vi "camera.vi"(0 "Camera configuration":string="{\n\t\"type\": \"Camera\",\n\t\"listen_port\": 8010,\n\t\"location\": {\n\t\t\"x\": 0.0,\n\t\t\"y\": 0.0,\n\t\t\"z\": 250.0\n\t},\n\t\"rotation\": {\n\t\t\"pitch\": 0.0,\n\t\t\"yaw\": 0.0,\n\t\t\"roll\": 0.0\n\t},\n\t\"stream_dimensions\": {\n\t\t\"x\": 512.0,\n\t\t\"y\": 512.0\n\t},\n \"dynamic_range\": 1.0,\n \"fov\": 60.0,\n \"camera_matrix\": [\n      [433.0, 0.0,   256.0],\n      [0.0,   433.0, 256.0],\n      [0.0,   0.0,   1.0]\n  ],\t\n \"min_shutter\": 0.0005,\n \"max_shutter\": 0.0014,\n \"motion_blur_bias\": 0.1,\n \"white_balance\": 0.0,\n \"white_balance_temp_offset\": 0,\n \"exposure_compensation\": -1.0,\n \"image_noise_bias\": 0.05,\n\t\"ray_tracing\": {\n\t\t\"enable_ray_tracing\": false\n\t},\n\t\"color_filter_array\": {\n\t\t\"use_cfa\": false,\n\t\t\"cfa\": \"rccc\"\n\t},\n\t\"channels\": \"bgra\",\n\t\"viewport\": {\n\t\t\"enable_viewport\": false,\n\t\t\"fullscreen\": false,\n\t\t\"monitor_name\": \"\",\n\t\t\"monitor_number\": 0,\n\t\t\"window_offset\": {\n\t\t\t\"x\": 32,\n\t\t\t\"y\": 32\n\t\t},\n\t\t\"window_size\": {\n\t\t\t\"x\": 0,\n\t\t\t\"y\": 0\n\t\t}\n\t},\n\t\"annotation\": {\n\t\t\"include_annotation\": false,\n\t\t\"desired_tags\": [\n\t\t\t\"traffic_sign\", \"vehicle\"\n\t\t],\n\t\t\"include_lanes\": true,\n\t\t\"lane_sampling_distance\": 15000.0,\n\t\t\"lane_sampling_frequency\": 100.0,\n\t\t\"lane_subsampling\": 10.0,\n\t\t\"far_plane\": 10000.0,\n\t\t\"include_tags\": true,\n\t\t\"include_obb\": false,\n\t\t\"cull_partial_frame\": false,\n\t\t\"debug_draw\": false\n\t},\n\t\"max_distance\": 50000.0,\n\t\"channel_depth\": 1\n}", 3 "error In":errorcluster) -> (4 "Camera configuration":string, 6 "Image":picture, 7 "Raw data":u8[](array[numeric]), 8 "Annotation Data":string, 9 "error out":errorcluster)   [LabVIEW 2019, in "Lib_Simx.lvlib"]
doc: "Configures and reads the data stream for a RGB Camera sensor and outputs a picture with the specified format in the stream dimensions."
uses:
  Lib_Simx.lvlib
  controls/Header.ctl
  tools/simx_common.vi
panel:
  out "Header":T1 {"game_time" format="%_10g"}
  in  "Show Annotation":bool
  in  "null connection":refnum<k5>
  in  "camera_connection":refnum<k5>
  # "Note: set annotation settings in camera configuration json"
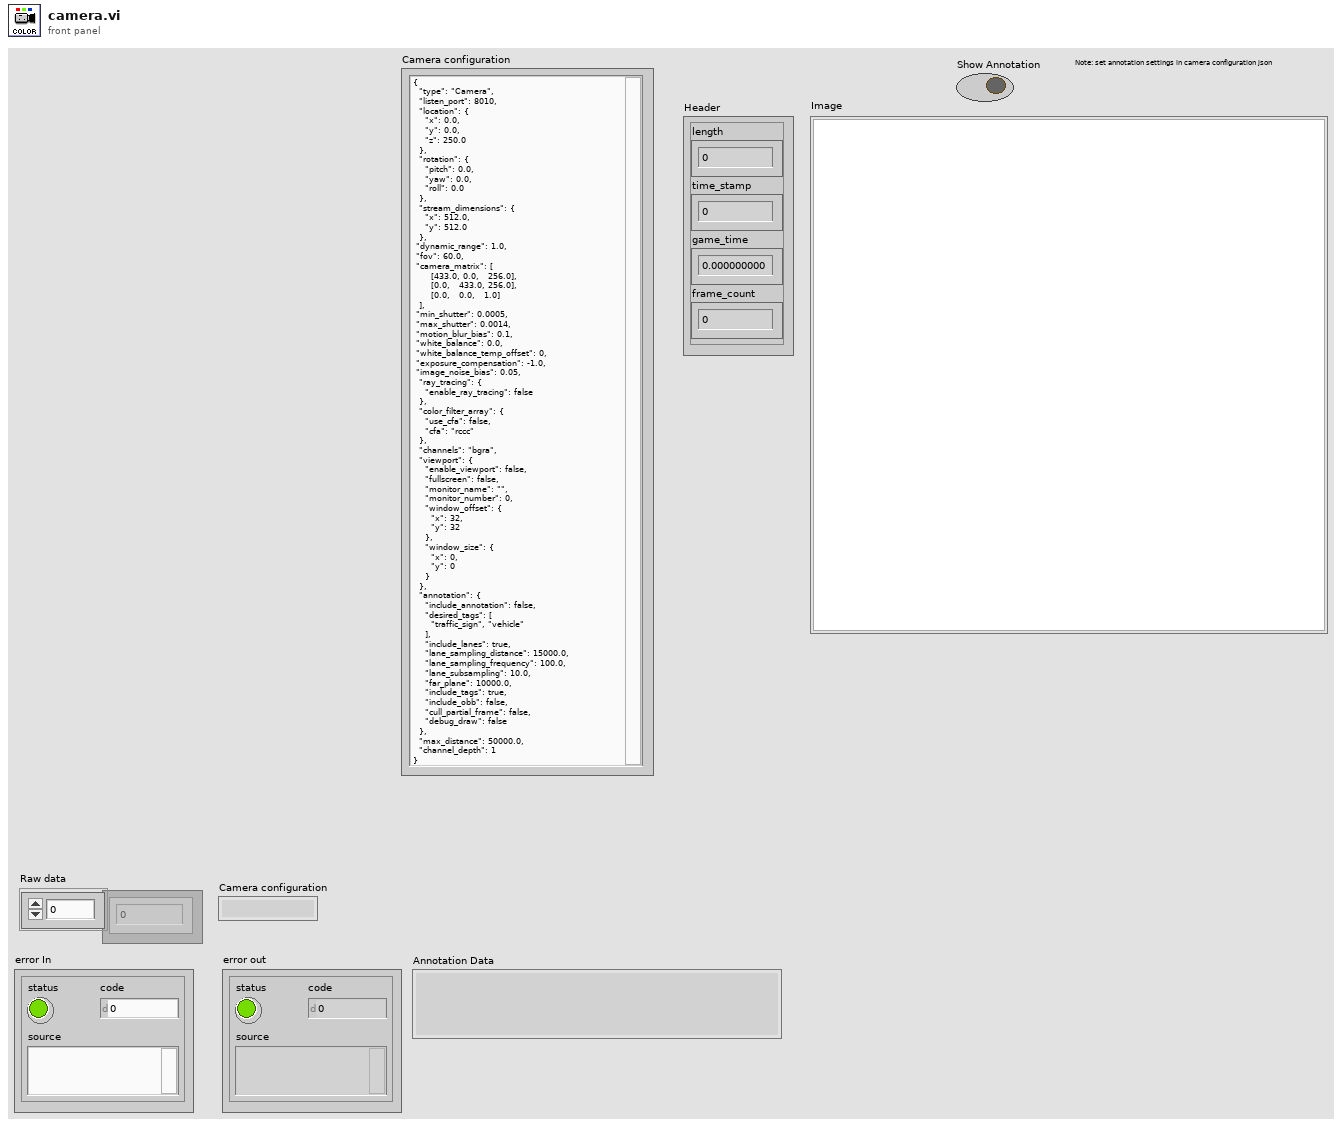
[diagram p1: front panel]
types:
  T1 = typedef "Lib_Simx.lvlib/Header.ctl" = cluster{"length":u32, "time_stamp":u32, "game_time":sgl, "frame_count":u32}
  T2 = typedef "Lib_Simx.lvlib/simx_connection.ctl" = cluster{"Config":T3, "Connections":T6, "Map":cluster{"lanes":cluster{"x":dbl[], "y":dbl[], "z":dbl[]}, "StartPosition":cluster{"start_points":T7, "StartRotation":dbl[], "StartLocation":dbl[]}, "Draw Map Size":T8, "DrawArea":cluster{"min_Y":dbl, "min_X":dbl, "Scale X":dbl, "Scale Y":dbl}, "Map":picture, "Map Geojson":string}}
  T3 = typedef "Lib_Simx.lvlib/config.ctl" = cluster{"Trajectory":T4, "Weather":T5}
  T4 = typedef "Lib_Simx.lvlib/trajectory.ctl" = cluster{"Number of frames":i32, "Frame number":i32, "Trajectory":string}
  T5 = typedef "Lib_Simx.lvlib/weather.ctl" = cluster{"id":string}
  T6 = typedef "Lib_Simx.lvlib/connections.ctl" = cluster{"Simulator Connection":refnum<k5>, "server_ip":string, "Port":i32, "Sensor connections":refnum<k5>[]}
  T7 = typedef "Lib_Simx.lvlib/start_points.ctl" = cluster{"locations":dbl[][], "rotations":dbl[][], "type":string[]}
  T8 = typedef "LVBoundsTypeDef.ctl" = cluster{"Width":u32, "Height":u32}
  T9 = typedef "Lib_Simx.lvlib/sensor_sample.ctl" = cluster{"Header":T1, "data out":string}
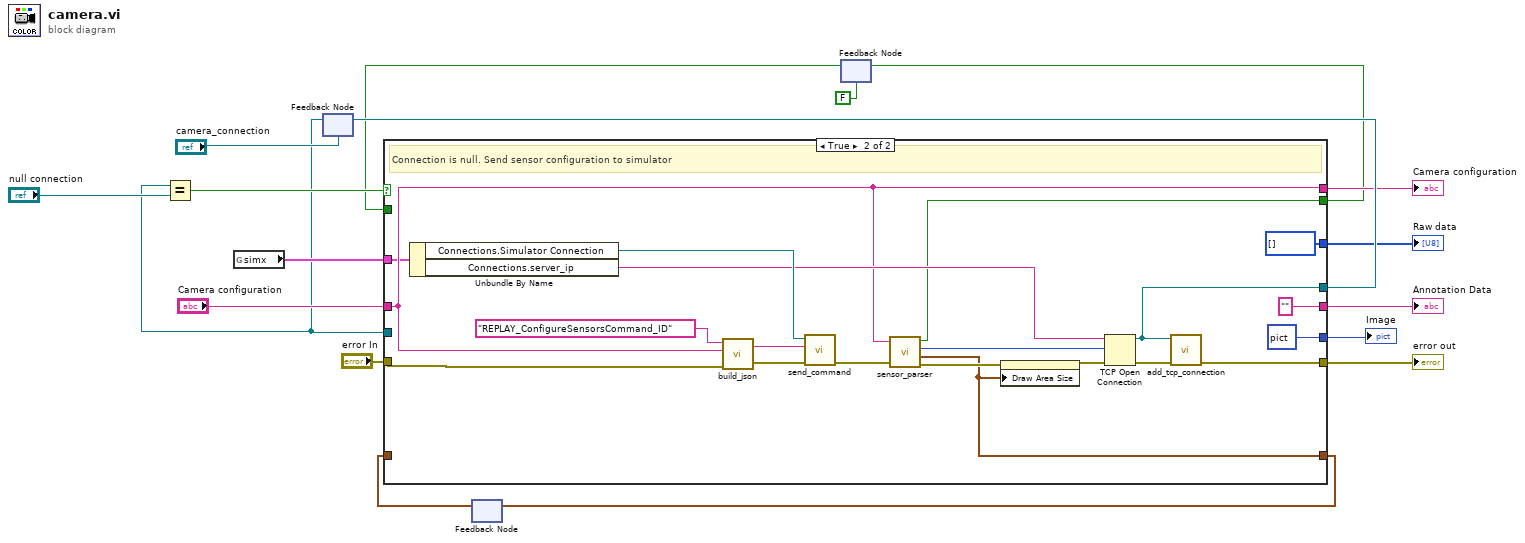
[diagram p0: block diagram]
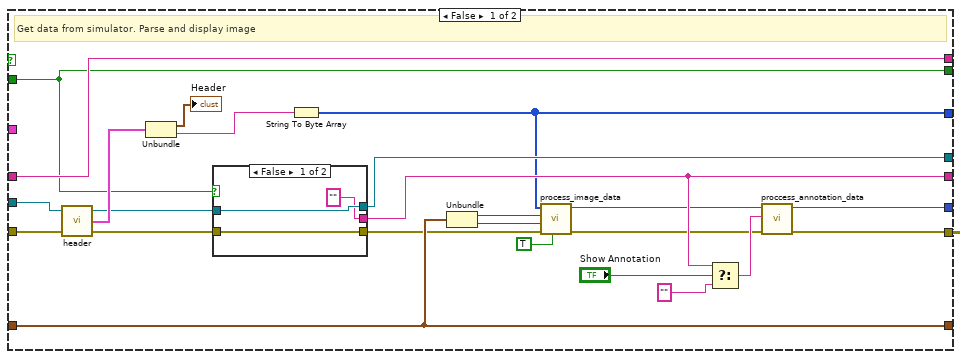
[diagram p2: hidden frame]
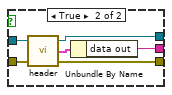
[diagram p3: hidden frame]
diagram:
  n1 = global read "simx_common.vi" "simx"() -> (w2:T2)
  n2 = feedback #1("camera_connection") -> (w1:refnum<k5>)
  n3 = Equal?(x=w1, y="null connection") -> (x = y?=w15:bool)
  n4 = feedback #2() -> (w10:cluster{"x dimension":i32, "y dimension":i32})  [unwired: 1 in]
  n5 = feedback #3(FALSE) -> (w4:bool)
  n6 = case shown="True" w15 {
    tunnel: [w35 w52] -> w13
    tunnel: "Camera configuration" -> [w37 w56]
    tunnel: [w27 w54] -> w16
    tunnel: w1 -> [w40 _]
    tunnel: "error In" -> [w39 w62]
    tunnel: w10 -> [w38 _]
    tunnel: [w34 picture data[5B] ("new picture")] -> w7
    tunnel: [w38 w59] -> w11
    tunnel: [w23 u8[] [] ("unsigned byte array")] -> w9
    tunnel: [w37 w56] -> w8
    tunnel: [w36 w58] -> w6
    tunnel: w4 -> [w36 _]
    tunnel: [w33 "" ("data out")] -> w3
    tunnel: w2 -> [_ w55]
    frame False {
      # "Get data from simulator. Parse and display image"
      n7 = call "header.vi"("error in"=w39, "TCP Network Connection in"=w40) -> ("error out"=w24:errorcluster, "Sensor sample"=w41:T9, "TCP Network Connection out"=w31:refnum<k5>)  [unwired: 1 in]
      n8 = Unbundle(w41) -> ("Header"=→"Header":T1, "data out"=w42:string)
      n9 = case shown="False" w36 {
        tunnel: w31 -> [w45 w51]
        tunnel: [w45 w50] -> w27
        tunnel: w24 -> [w43 w49]
        tunnel: ["" ("data out") w47] -> w33
        tunnel: [w43 w46] -> w26
        frame False {
        }
        frame True {
          n10 = call "header.vi"("error in"=w49, "TCP Network Connection in"=w51) -> ("error out"=w46:errorcluster, "Sensor sample"=w48:T9, "TCP Network Connection out"=w50:refnum<k5>)  [unwired: 1 in]
          n11 = Unbundle By Name(w48) -> ("data out"=w47:string)
        }
      }
      n12 = String To Byte Array(string=w42) -> (unsigned byte array=w23:u8[])
      n13 = Unbundle(w38) -> ("x dimension"=w22:i32, "y dimension"=w21:i32)
      n14 = call "process_image_data.vi"("RGBA"=TRUE, "error in"=w26, "y"=w21, "x"=w22, "Raw data"=w23) -> ("error out"=w25:errorcluster, "Image"=w20:picture)  [unwired: 3 in]
      n15 = Select(t=w33, s="Show Annotation", f="") -> (s? t:f=w28:string)
      n16 = call "proccess_annotation_data.vi"("error in"=w25, "Annotation Data"=w28, "Image in"=w20) -> ("error out"=w35:errorcluster, "Image out"=w34:picture)  [unwired: 2 in, 1 out]
    }
    frame True {
      # "Connection is null. Send sensor configuration to simulator"
      n17 = Unbundle By Name(w55) -> ("Connections.Simulator Connection"=w65:refnum<k5>, "Connections.server_ip"=w63:string)
      n18 = call "build_json.vi"("error in"=w62, "Message"=w56, "Command_ID"="REPLAY_ConfigureSensorsCommand_ID") -> ("error out"=w69:errorcluster, "JSON Out"=w70:string)  [unwired: 1 in]
      n19 = call "send_command.vi"("error in"=w69, "JSON Command"=w70, "TCP Network Connection in"=w65) -> ("error out"=w61:errorcluster)  [unwired: 1 in, 3 out]
      n20 = call "sensor_parser.vi"("Sensor configuration"=w56, "error in"=w61) -> ("include_annotation"=w58:bool, "Port out"=w57:u16, "Stream dimensions"=w59:cluster{"x dimension":i32, "y dimension":i32}, "error out"=w60:errorcluster)  [unwired: 1 in]
      n21 = property on="Image" class="Pict"(error in=w60, "Draw Area Size"=w59) -> (error out=w64:errorcluster)  [unwired: 1 in, 1 out]
      n22 = TCP Open Connection(address=w63, remote port or service name=w57, error in (no error)=w64) -> (connection ID=w54:refnum<k5>, error out=w53:errorcluster)  [unwired: 2 in]
      n23 = call "add_tcp_connection.vi"("error in"=w53, "Sensor connection"=w54) -> ("error out"=w52:errorcluster)  [unwired: 5 in]
    }
  }
  "error out" <- w13
  "Image" <- w7
  "Raw data" <- w9
  "Camera configuration" <- w8
  "Annotation Data" <- w3
  n24 = feedback-in #1(w16) -> ()
  n25 = feedback-in #2(w11) -> ()
  n26 = feedback-in #3(w6) -> ()
